vi "checkPauseTimeElapsed.vi"(8 "error in (no error)":errorcluster, 11 "Model in":refnum<class "Model.lvclass">) -> (0 "error out":errorcluster, 2 "pauseTimeHasElapsedIsTrue":bool, 3 "Model out":refnum<class "Model.lvclass">)   [LabVIEW 2013, in "Model.lvclass"]
uses:
  Model.lvclass
  Model.lvclass/Model.ctl
  UserEvents/UserEvents.lvclass/UserEvents.ctl
  ApplicationElements/TestMonitor/TestMonitor.lvclass
  UserEvents/UserEvents.lvclass
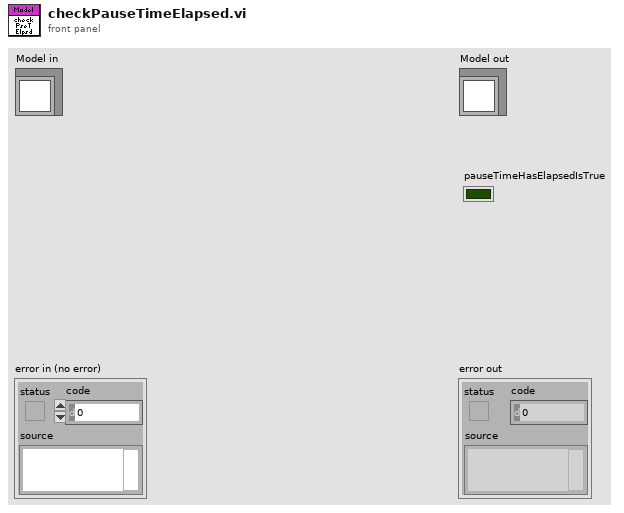
[diagram p1: front panel]
types:
  T1 = typedef "AITDTTypedefs.lvlib/PubDataEvents.ctl" = cluster{"State":refnum<user-event>, "ErrorCode":refnum<user-event>, "OutputData":refnum<user-event>, "InputData":refnum<user-event>, "TestStatus":refnum<user-event>, "LogPath":refnum<user-event>, "TemperatureSetpointRequest":refnum<user-event>, "TemperatureSettling":refnum<user-event>, "WaitTimeStatus":refnum<user-event>}
  T2 = typedef "AITDTTypedefs.lvlib/WaitTimeStatus.ctl" = cluster{"Required Wait Time":dbl[unit], "Elapsed Wait Time":dbl[unit]}
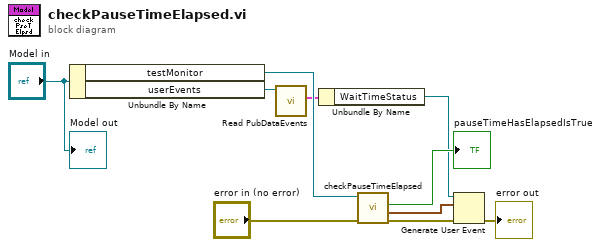
[diagram p0: block diagram]
diagram:
  n1 = Unbundle By Name("Model in") -> ("testMonitor"=w9:refnum<class "TestMonitor.lvclass">, "userEvents"=w6:refnum<class "UserEvents.lvclass">)
  n2 = call "Read PubDataEvents.vi"("UserEvents in"=w6) -> ("PubDataEvents"=w4:T1)  [unwired: 9 in, 1 out]
  n3 = Unbundle By Name(w4) -> ("WaitTimeStatus"=w5:refnum<user-event>)
  n4 = call "checkPauseTimeElapsed.vi"("error in (no error)"="error in (no error)", "TestMonitor in"=w9) -> ("error out"=w2:errorcluster, "Wait Time Status"=w3:T2, "pauseTimeElapsedIsTrue"=→"pauseTimeHasElapsedIsTrue":bool)  [unwired: 6 in, 1 out]
  n5 = Generate User Event(user event=w5, event data cluster=w3, error in=w2) -> (error out=→"error out":errorcluster)  [unwired: 1 in, 1 out]
  "Model out" <- "Model in"
